vi "UTILITY This VIs Path.vi"(0 "path":path, 11 "error in (no error)":errorcluster) -> (2 "Folder Path":path, 3 "Robocopy Path":string, 4 "Application:Kind":T2(ring), 6 "current path":path, 8 "File Version Info":string, 10 "FileVersionInfo Out":T1, 15 "error out":errorcluster)   [LabVIEW 2019]
uses:
  <vilib>/Platform/fileVersionInfo.llb/FileVersionInformation.ctl
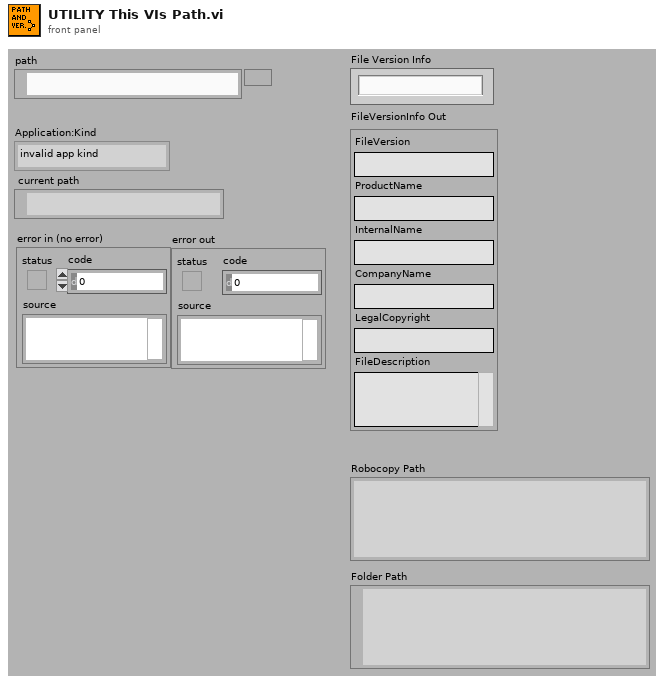
[diagram p1: front panel]
types:
  T1 = typedef "FileVersionInformation.ctl" = cluster{"FileVersion":string, "ProductName":string, "InternalName":string, "CompanyName":string, "LegalCopyright":string, "FileDescription":string}
  T2 = enum32{"invalid app kind", "Development System", "Run Time System", "Student Edition", "Embedded LabVIEW", "Evaluation", "Custom"}
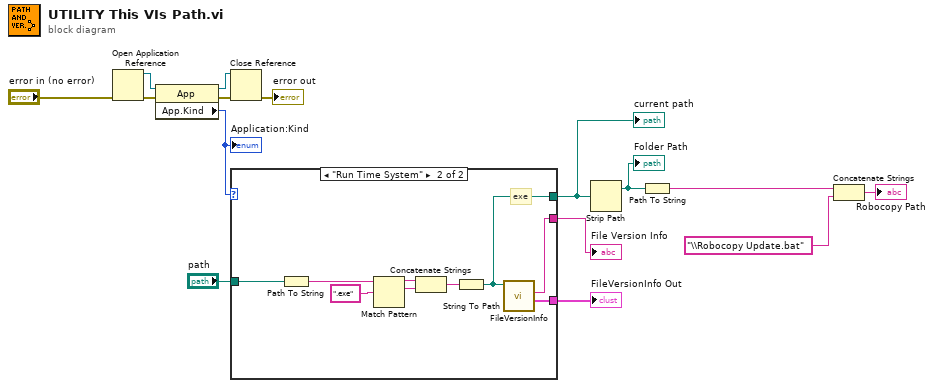
[diagram p0: block diagram]
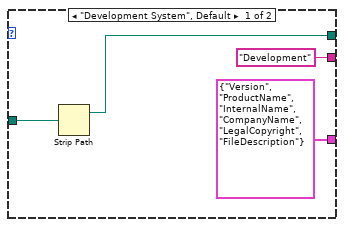
[diagram p2: hidden frame]
diagram:
  n1 = Open Application Reference(8:"error in (no error)") -> (0:w9:errorcluster, 3:w14:refnum<vi>)  [unwired: 3 in]
  n2 = property class="App"(reference=w14, error in=w9) -> (reference out=w12:refnum<vi>, error out=w13:errorcluster, "App.Kind"=w15:T2)
  "Application:Kind" <- w15
  n3 = Close Reference(reference=w12, error in (no error)=w13) -> (error out=→"error out":errorcluster)
  n4 = case shown="\"Run Time System\"" w15 {
    tunnel: [w19 w20] -> w2
    tunnel: "path" -> [w18 w26]
    tunnel: ["Development" ("File Version Info") w28] -> w11
    tunnel: [T1 {"FileVersion"="Version", "ProductName"="ProductName", "InternalName"="InternalName", "CompanyName"="CompanyName", "LegalCopyright"="LegalCopyright", "FileDescription"="FileDescription"} ("FileVersionInfo Out") w27] -> w6
    frame "Development System", Default {
      n5 = Strip Path(path=w18) -> (stripped path=w19:path)  [unwired: 1 out]
    }
    frame "Run Time System" {
      # "exe"
      n6 = Path To String(path=w26) -> (string=w25:string)
      n7 = Match Pattern(string=w25, regular expression=".exe") -> (before substring=w23:string, match substring=w22:string)  [unwired: 1 in, 2 out]
      n8 = Concatenate Strings(w23, w22) -> (w21:string)
      n9 = String To Path(string=w21) -> (path=w20:path)
      n10 = call <vilib>:"FileVersionInfo.vi"("Application Path in"=w20) -> ("FileVersionInfo Out"=w27:T1, "File Version Info"=w28:string)  [unwired: 7 in, 2 out]
    }
  }
  "current path" <- w2
  "File Version Info" <- w11
  "FileVersionInfo Out" <- w6
  n11 = Strip Path(path=w2) -> (stripped path=w3:path)  [unwired: 1 out]
  "Folder Path" <- w3
  n12 = Path To String(path=w3) -> (string=w4:string)
  n13 = Concatenate Strings(w4, "\\Robocopy Update.bat" ("command line")) -> (→"Robocopy Path":string)
